vi "Maybe Add Pending Fixed Value.vi"(11 "Pattern Parser In":T1) -> (0 "error out":errorcluster, 3 "Pattern Parser":T1)   [LabVIEW 2020, in "Stream.lvlib" / "URLPattern.lvclass"]
uses:
  URLPattern.lvclass
  Pattern Parser.ctl
  Token.ctl
  Token Type.ctl
  Pattern Part.ctl
  Pattern Part Type.ctl
  Pattern Part Modifier.ctl
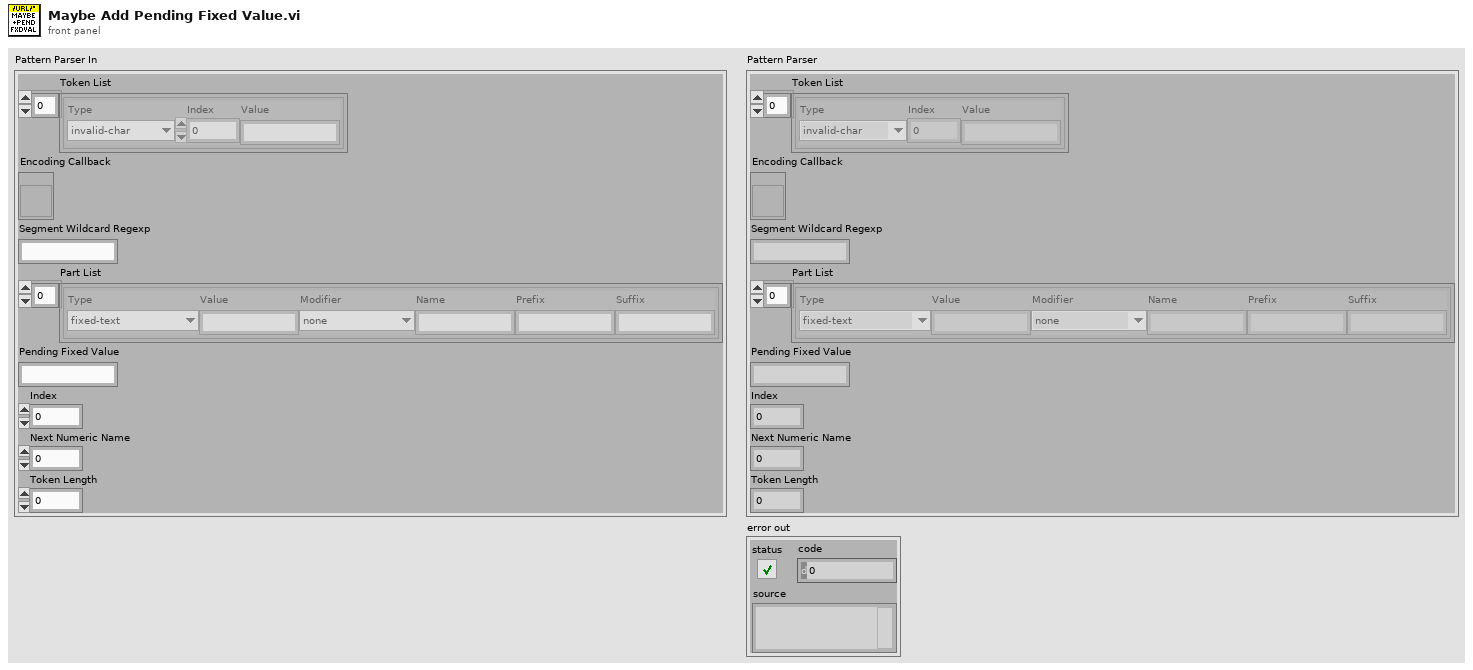
[diagram p1: front panel]
types:
  T1 = typedef "Stream.lvlib/URLPattern.lvclass/Pattern Parser.ctl" = cluster{"Token List":T2[], "Encoding Callback":refnum<vi>, "Segment Wildcard Regexp":string, "Part List":T4[], "Pending Fixed Value":string, "Index":i32, "Next Numeric Name":i32, "Token Length":i32}
  T2 = typedef "Stream.lvlib/URLPattern.lvclass/Token.ctl" = cluster{"Type":T3, "Index":i32, "Value":string}
  T3 = typedef "Stream.lvlib/URLPattern.lvclass/Token Type.ctl" = enum16{"invalid-char", "open", "close", "regexp", "name", "char", "escaped-char", "other-modifier", "asterisk", "end"}
  T4 = typedef "Stream.lvlib/URLPattern.lvclass/Pattern Part.ctl" = cluster{"Type":T5, "Value":string, "Modifier":T6, "Name":string, "Prefix":string, "Suffix":string}
  T5 = typedef "Stream.lvlib/URLPattern.lvclass/Pattern Part Type.ctl" = enum16{"fixed-text", "regexp", "segment-wildcard", "full-wildcard"}
  T6 = typedef "Stream.lvlib/URLPattern.lvclass/Pattern Part Modifier.ctl" = enum16{"none", "optional", "zero-or-more", "one-or-more"}
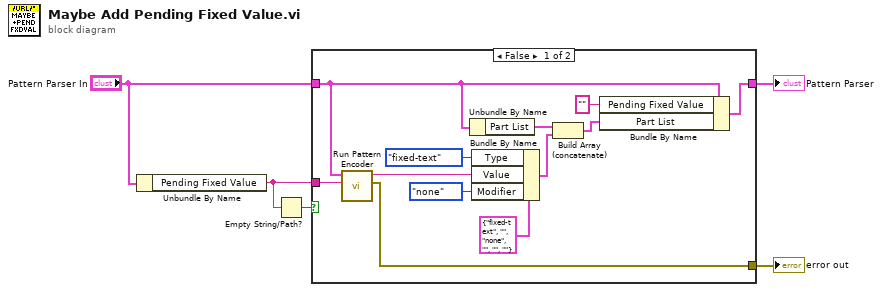
[diagram p0: block diagram]
diagram:
  n1 = Unbundle By Name("Pattern Parser In") -> ("Pending Fixed Value"=w4:string)
  n2 = Empty String/Path?(string/path=w4) -> (empty?=w5:bool)
  n3 = case shown="False" w5 {
    tunnel: w4 -> [w9 _]
    tunnel: "Pattern Parser In" -> [w8 w18]
    tunnel: [w14 w18] -> w2
    tunnel: [w6 _] -> w1
    frame False {
      n4 = call "Run Pattern Encoder.vi"("Input"=w9, "Pattern Parser"=w8) -> ("error out"=w6:errorcluster, "Encoded"=w7:string)  [unwired: 8 in]
      n5 = Unbundle By Name(w8) -> ("Part List"=w12:T4[])
      n6 = Bundle By Name(cluster=T4 {"Type"=enum."fixed-text", "Value"="", "Modifier"=enum."none", "Name"="", "Prefix"="", "Suffix"=""} ("Pattern Part"), "Type"=Pattern_Part_Type."fixed-text", "Value"=w7, "Modifier"=Pattern_Part_Modifier."none") -> (w11:T4)
      n7 = Build Array (concatenate)(w12, w11) -> (w10:T4[])
      n8 = Bundle By Name(cluster=w8, "Pending Fixed Value"="", "Part List"=w10) -> (w14:T1)
    }
    frame True {
    }
  }
  "Pattern Parser" <- w2
  "error out" <- w1
